vi "_getFiles.vi"(7 "Selected path":path) -> (3 "Import files":string[](array[string]))   [LabVIEW 2019, in "SEECD System Explorer.lvlib"]
uses:
  SEECD System Explorer.lvlib
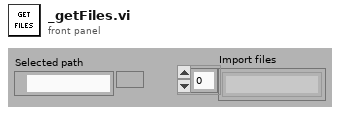
[diagram p1: front panel]
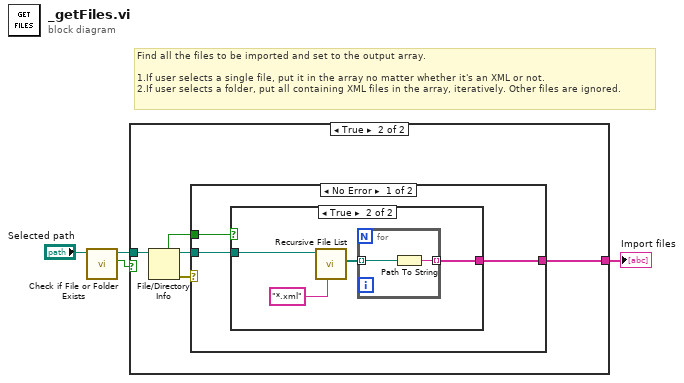
[diagram p0: block diagram]
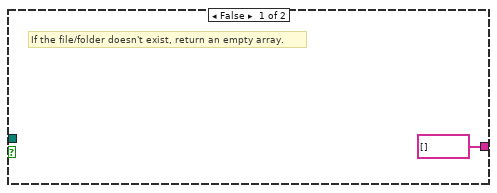
[diagram p2: hidden frame]
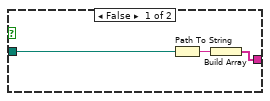
[diagram p3: hidden frame]
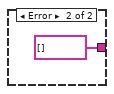
[diagram p4: hidden frame]
diagram:
  # "Find all the files to be imported and set to the output array.\n\n1.If user selects a single file, put it in the array no matter whether it's an XML or not.\n2.If user selects a folder, put all containing XML files in the array, iteratively. Other files are ignored."
  n1 = call <vilib>:"Check if File or Folder Exists.vi"("path"="Selected path") -> ("file or folder exists?"=w4:bool, "dup path"=w2:path)  [unwired: 1 in, 8 out]
  n2 = case shown="True" w4 {
    tunnel: w2 -> [_ w10]
    tunnel: [string[] [] w7] -> w1
    frame False {
      # "If the file/folder doesn't exist, return an empty array."
    }
    frame True {
      n3 = File/Directory Info(path=w10) -> (path out=w8:path, directory=w9:bool, error out=w6:errorcluster)  [unwired: 1 in, 4 out]
      n4 = case shown="No Error" w6 {
        tunnel: w9 -> [w13 _]
        tunnel: w8 -> [w12 _]
        tunnel: [w11 string[] []] -> w7
        frame No Error {
          n5 = case shown="True" w13 {
            tunnel: w12 -> [w16 w20]
            tunnel: [w14 w17] -> w11
            frame False {
              n6 = Path To String(path=w16) -> (string=w15:string)
              n7 = Build Array(w15) -> (w14:string[])
            }
            frame True {
              n8 = call <vilib>:"Recursive File List.vi"("pattern"="*.xml", "Folder Path"=w20) -> ("All Files in Dir"=w19:path[])  [unwired: 2 in, 7 out]
              n9 = for {
                tunnel: w19 -> [w22] mode=indexing
                tunnel: [w21] -> w17 mode=indexing
                n10 = Path To String(path=w22) -> (string=w21:string)
              }
            }
          }
        }
        frame Error {
        }
      }
    }
  }
  "Import files" <- w1
